vi "RateOfChangeLM35.vi"(10 "Last Reading":dbl[](array[numeric]), 11 "Current Reading":dbl[](array[numeric])) -> (3 "Rate of Change Output":dynamicdata(waveform))   [LabVIEW 2020]
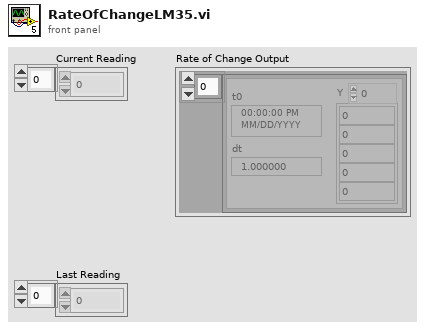
[diagram p1: front panel]
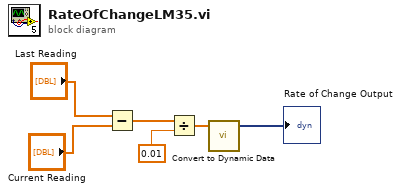
[diagram p0: block diagram]
diagram:
  n1 = Subtract(x="Last Reading", y="Current Reading") -> (x-y=w3:dbl[])
  n2 = Divide(x=w3, y=0.01) -> (x/y=w5:dbl[])
  n3 = call "Convert to Dynamic Data"("Array"=w5) -> ("Dynamic Data Type"=→"Rate of Change Output":dynamicdata)  [unwired: 3 in]
